vi "Create From String.vi"(8 "error in":errorcluster, 10 "Input String":string) -> (0 "error out":errorcluster, 3 "Vec3d out":refnum<class "Vec3d Class.lvclass">)   [LabVIEW 2011, in "Vec3d Class.lvclass"]
uses:
  Vec3d Class.lvclass
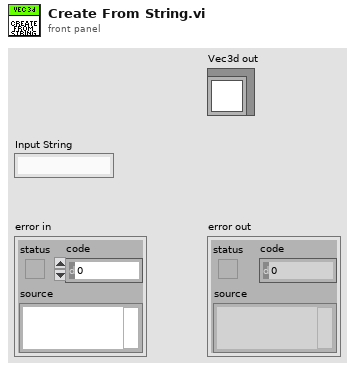
[diagram p1: front panel]
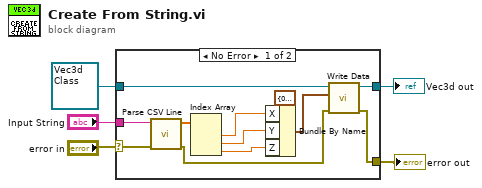
[diagram p0: block diagram]
diagram:
  n1 = case shown="No Error" "error in" {
    selector: "error in" -> [w13 w19]
    tunnel: [w15 w19] -> w2
    tunnel: [w16 w18] -> w5
    tunnel: refnum<class "Vec3d Class.lvclass"> refnum ("Vec3d Class in") -> [w17 w18]
    tunnel: "Input String" -> [w14 _]
    frame No Error {
      n2 = call "Parse CSV Line.vi"("error in"=w13, "Input String"=w14) -> ("error out"=w11:errorcluster, "values"=w9:dbl[])  [unwired: 8 in]
      n3 = Index Array(array=w9) -> (element #1=w8:dbl, element #2=w7:dbl, element #3=w6:dbl)  [unwired: 3 in]
      n4 = Bundle By Name(cluster=cluster{"X":dbl, "Y":dbl, "Z":dbl} {"X"=0.0, "Y"=0.0, "Z"=0.0} ("Data"), "X"=w8, "Y"=w7, "Z"=w6) -> (w10:cluster{"X":dbl, "Y":dbl, "Z":dbl})
      n5 = call-dynamic "Write Data.vi"("error in (no error)"=w11, "Data"=w10, "Vec3d Class in"=w17) -> ("error out"=w15:errorcluster, "Vec3d Class out"=w16:refnum<class "Vec3d Class.lvclass">)  [unwired: 7 in]
    }
    frame Error {
    }
  }
  "error out" <- w2
  "Vec3d out" <- w5
